vi "StopMotion.vi"(8 "error in (no error)":errorcluster, 9 "SendMessage":refnum<class "SendMessage.lvclass">, 11 "sub-systems in":refnum<class "sub-systems.lvclass">) -> (0 "error out":errorcluster, 3 "sub-systems out":refnum<class "sub-systems.lvclass">)   [LabVIEW 2018, in "sub-systems.lvclass"]
uses:
  sub-systems.lvclass
  SendMessage/SendMessage.lvclass
  VSMx2/VXMx2.lvclass
panel:
  # "has a"
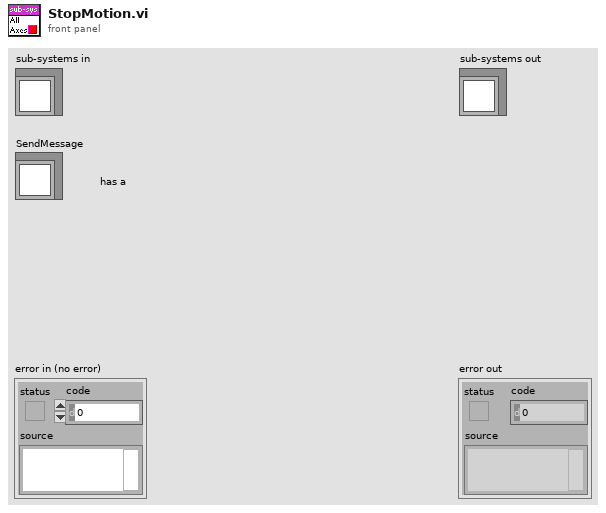
[diagram p1: front panel]
types:
  T1 = cluster{"mmWaveName":string, "Sub-syst":i32, "Axis":string}[]
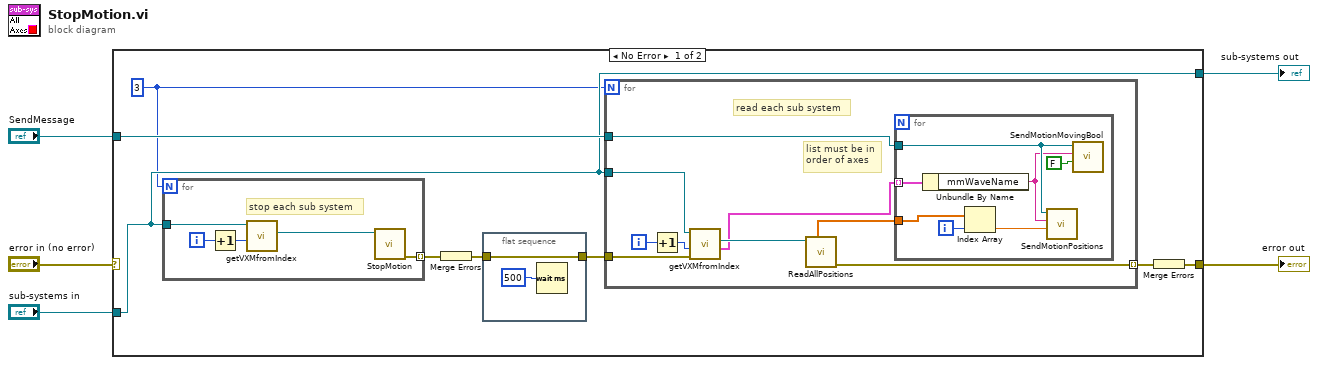
[diagram p0: block diagram]
diagram:
  n1 = case shown="No Error" "error in (no error)" {
    selector: "error in (no error)" -> [_ w38]
    tunnel: [w7 w38] -> w4
    tunnel: [w9 w37] -> w2
    tunnel: "sub-systems in" -> [w9 w37]
    tunnel: "SendMessage" -> [w13 _]
    frame No Error {
      w6 = 3
      n2 = for {
        N: w6 -> [_]
        tunnel: [w36] -> w12 mode=indexing
        tunnel: w9 -> [w35]
        i -> [w34]
        # "stop each sub system"
        n3 = Increment(x=w34) -> (x+1=w32:i32)
        n4 = call "getVXMfromIndex.vi"("Subsystem 1, 2, 3"=w32, "sub-systems in"=w35) -> ("VXMx2 out"=w33:refnum<class "VXMx2.lvclass">)  [unwired: 5 in, 4 out]
        n5 = call "StopMotion.vi"("VXMx2 in"=w33) -> ("error out"=w36:errorcluster)  [unwired: 8 in, 2 out]
      }
      n6 = Merge Errors(w12) -> (w11:errorcluster)
      n7 = flat-sequence {
        tunnel: [w14] -> w10
        tunnel: w11 -> [w14]
        frame #0 {
          n8 = Wait (ms)(milliseconds to wait=u32 500) -> ()  [unwired: 1 out]
        }
      }
      n9 = for {
        N: w6 -> [_]
        tunnel: [w24] -> w8 mode=indexing
        tunnel: w9 -> [w23]
        tunnel: w13 -> [w19]
        tunnel: w10 -> [w16]
        i -> [w22]
        # "list must be in\norder of axes"
        # "read each sub system"
        n10 = Increment(x=w22) -> (x+1=w17:i32)
        n11 = call "getVXMfromIndex.vi"("error in (no error)"=w16, "Subsystem 1, 2, 3"=w17, "sub-systems in"=w23) -> ("All Axes this subsystem"=w20:T1, "VXMx2 out"=w21:refnum<class "VXMx2.lvclass">)  [unwired: 4 in, 3 out]
        n12 = call "ReadAllPositions.vi"("VXMx2 in"=w21) -> ("error out"=w24:errorcluster, "All Positions, eng units"=w18:dbl[])  [unwired: 3 in, 6 out]
        n13 = for {
          tunnel: w20 -> [w29] mode=indexing
          tunnel: w19 -> [w30]
          tunnel: w18 -> [w28]
          i -> [w27]
          n14 = Unbundle By Name(w29) -> ("mmWaveName"=w25:string)
          n15 = Index Array(array=w28, index=w27) -> (element=w26:dbl)
          n16 = call "SendMotionPositions.vi"("Axis Position, eng."=w26, "mmWave Axis Name"=w25, "SendMessage in"=w30) -> ()  [unwired: 7 in, 2 out]
          n17 = call "SendMotionMovingBool.vi"("Axis True= Moving"=FALSE, "mmWave Axis Name"=w25, "SendMessage in"=w30) -> ()  [unwired: 7 in, 2 out]
        }
      }
      n18 = Merge Errors(w8) -> (w7:errorcluster)
    }
    frame Error {
    }
  }
  "error out" <- w4
  "sub-systems out" <- w2
